vi "SwerveChooseCenter.vi"(6 "Defensive Driving Trigger":bool, 8 "Joystick Y":dbl, 9 "Joystick X":dbl) -> (2 "Cy (in)":dbl, 3 "Cx (in)":dbl)   [LabVIEW 2020]
doc: "This VI chooses a corner of the robot to pivot about during evasive manuervers based on the driver's current joystick commands."
uses:
  9a94878a-4914-4fba-839a-7657b048eec0.vi
  GlobalDrivebase.vi
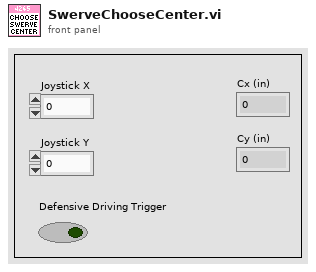
[diagram p1: front panel]
types:
  T1 = enum16{"Center", "Module 0", "Module 1", "Module 2", "Module 3"}
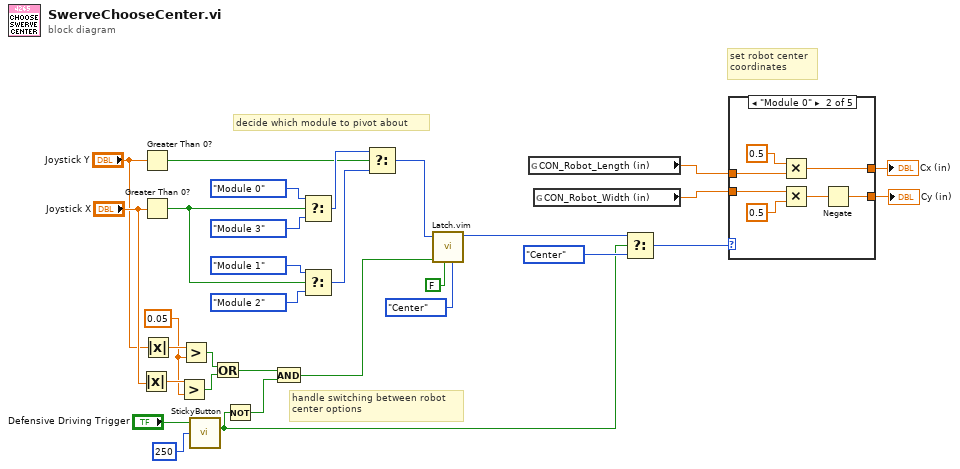
[diagram p0: block diagram]
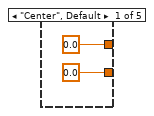
[diagram p2: hidden frame]
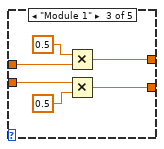
[diagram p3: hidden frame]
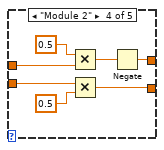
[diagram p4: hidden frame]
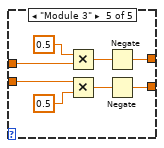
[diagram p5: hidden frame]
diagram:
  w14 = 0.05 ("y")
  # "handle switching between robot\ncenter options"
  # "decide which module to pivot about"
  # "set robot center \ncoordinates"
  n1 = Absolute Value(x="Joystick X") -> (abs(x)=w15:dbl)
  n2 = Greater Than 0?(x="Joystick Y") -> (x > 0?=w28:bool)
  n3 = Greater Than 0?(x="Joystick X") -> (x > 0?=w30:bool)
  n4 = Absolute Value(x="Joystick Y") -> (abs(x)=w16:dbl)
  n5 = Greater?(x=w15, y=w14) -> (0:w13:bool)
  n6 = Greater?(x=w16, y=w14) -> (0:w12:bool)
  n7 = call "StickyButton.vi"("Time threshold (ms)"=u32 250, "Button Input"="Defensive Driving Trigger") -> ("Sticky Button"=w1:bool)  [unwired: 1 in]
  n8 = Or(x=w12, y=w13) -> (x .or. y?=w11:bool)
  n9 = Not(x=w1) -> (.not. x?=w10:bool)
  n10 = And(x=w11, y=w10) -> (x .and. y?=w9:bool)
  n11 = Select(t=T1."Module 0", s=w30, f=T1."Module 3") -> (s? t:f=w29:T1)
  n12 = Select(t=T1."Module 1", s=w30, f=T1."Module 2") -> (s? t:f=w31:T1)
  n13 = Select(t=w29, s=w28, f=w31) -> (s? t:f=w8:T1)
  n14 = call "Latch.vim"("Default Value"=T1."Center", "Reset"=FALSE, "Latch Signal"=w9, "Latch Value"=w8) -> ("Latched"=w7:T1)  [unwired: 7 in]
  n15 = global read "GlobalDrivebase.vi" "CON_Robot_Length (in)"() -> (w5:dbl)
  n16 = global read "GlobalDrivebase.vi" "CON_Robot_Width (in)"() -> (w4:dbl)
  n17 = Select(t=w7, s=w1, f=T1."Center") -> (s? t:f=w6:T1)
  n18 = case shown="\"Module 0\"" w6 {
    tunnel: [0.0 w39 w42 w48 w55] -> w20
    tunnel: [0.0 w34 w41 w47 w54] -> w19
    tunnel: w5 -> [_ w40 w44 w51 w59]
    tunnel: w4 -> [_ w37 w43 w50 w58]
    frame "Center", Default {
    }
    frame "Module 0" {
      n19 = Multiply(x=0.5, y=w40) -> (x*y=w39:dbl)
      n20 = Multiply(x=w37, y=0.5) -> (x*y=w36:dbl)
      n21 = Negate(x=w36) -> (-x=w34:dbl)
    }
    frame "Module 1" {
      n22 = Multiply(x=0.5, y=w44) -> (x*y=w42:dbl)
      n23 = Multiply(x=w43, y=0.5) -> (x*y=w41:dbl)
    }
    frame "Module 2" {
      n24 = Multiply(x=0.5, y=w51) -> (x*y=w49:dbl)
      n25 = Multiply(x=w50, y=0.5) -> (x*y=w47:dbl)
      n26 = Negate(x=w49) -> (-x=w48:dbl)
    }
    frame "Module 3" {
      n27 = Multiply(x=0.5, y=w59) -> (x*y=w57:dbl)
      n28 = Multiply(x=w58, y=0.5) -> (x*y=w56:dbl)
      n29 = Negate(x=w57) -> (-x=w55:dbl)
      n30 = Negate(x=w56) -> (-x=w54:dbl)
    }
  }
  "Cx (in)" <- w20
  "Cy (in)" <- w19
